vi "Xbox Controller Worker.vi"(8 "Error In":errorcluster, 10 "Events":T2, 11 "Xbox One Controller Ref":T1={"Controller Ref"=refnum, "Event Refnum"=refnum, "Worker Ref"=refnum}) -> (0 "Error Out":errorcluster)   [LabVIEW 2011, in "LVH-Xbox-One-Controller.lvlib"]
uses:
  LVH-Xbox-One-Controller.lvlib
  Type Defs/Events.ctl
  Type Defs/Xbox One Controller Ref.ctl
  Type Defs/Indicators/All Buttons Visual.ctl
  Type Defs/Indicators/A.ctl
  Type Defs/Indicators/B.ctl
  Type Defs/Indicators/X.ctl
  Type Defs/Indicators/Y.ctl
  Type Defs/Indicators/Left Bumper.ctl
  Type Defs/Indicators/Right Bumper.ctl
  Type Defs/Indicators/View.ctl
  Type Defs/Indicators/Menu.ctl
  Type Defs/Indicators/Thumbstick.ctl
  <vilib>/Utility/inputDevices.llb/joystickAcquire.vi
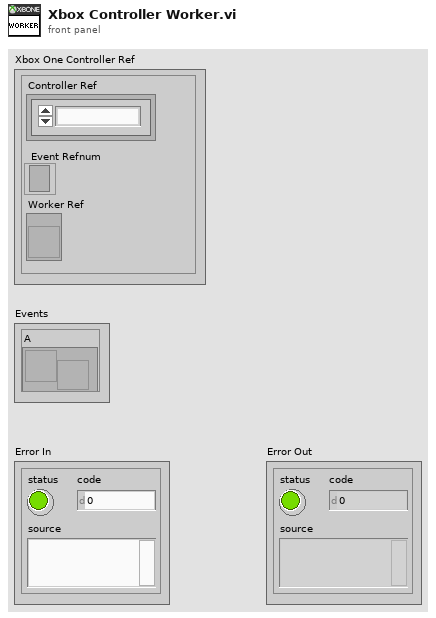
[diagram p1: front panel]
types:
  T1 = typedef "LVH-Xbox-One-Controller.lvlib/Xbox One Controller Ref.ctl" = cluster{"Controller Ref":refnum<k1>, "Event Refnum":refnum<event-registration>, "Worker Ref":refnum<vi>}
  T2 = typedef "LVH-Xbox-One-Controller.lvlib/Events.ctl" = cluster{"A":refnum<user-event>, "B":refnum<user-event>, "X":refnum<user-event>, "Y":refnum<user-event>, "Left Bumper":refnum<user-event>, "Right Bumper":refnum<user-event>, "View":refnum<user-event>, "Menu":refnum<user-event>, "Left Stick":refnum<user-event>, "Right Stick":refnum<user-event>}
  T3 = typedef "LVH-Xbox-One-Controller.lvlib/All Buttons Visual.ctl" = cluster{"A":T4, "B":T5, "X":T6, "Y":T7, "Left Bumper":T8, "Right Bumper":T9, "View Button":T10, "Menu Button":T11, "Left Stick":T12, "Right Stick":T12}
  T4 = typedef "LVH-Xbox-One-Controller.lvlib/A.ctl" = bool
  T5 = typedef "LVH-Xbox-One-Controller.lvlib/B.ctl" = bool
  T6 = typedef "LVH-Xbox-One-Controller.lvlib/X.ctl" = bool
  T7 = typedef "LVH-Xbox-One-Controller.lvlib/Y.ctl" = bool
  T8 = typedef "LVH-Xbox-One-Controller.lvlib/Left Bumper.ctl" = bool
  T9 = typedef "LVH-Xbox-One-Controller.lvlib/Right Bumper.ctl" = bool
  T10 = typedef "LVH-Xbox-One-Controller.lvlib/View.ctl" = bool
  T11 = typedef "LVH-Xbox-One-Controller.lvlib/Menu.ctl" = bool
  T12 = typedef "LVH-Xbox-One-Controller.lvlib/Thumbstick.ctl" = bool
  T13 = cluster{"button 1":bool, "button 2":bool, "button 3":bool, "button 4":bool, "button 5":bool, "button 6":bool, "button 7":bool, "button 8":bool, "button 9":bool, "button 10":bool, "button 11":bool, "button 12":bool, "button 13":bool, "button 14":bool, "button 15":bool, "button 16":bool, "button 17":bool, "button 18":bool, "button 19":bool, "button 20":bool, "button 21":bool, "button 22":bool, "button 23":bool, "button 24":bool, "button 25":bool, "button 26":bool, "button 27":bool, "button 28":bool, "button 29":bool, "button 30":bool, "button 31":bool, "button 32":bool}
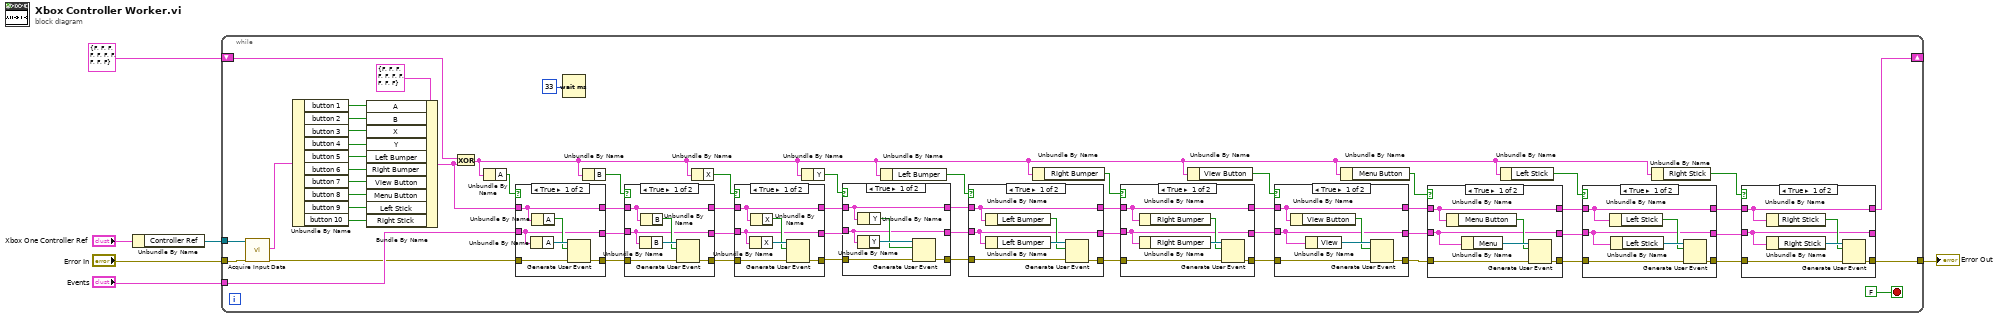
[diagram p0: block diagram]
diagram:
  n1 = Unbundle By Name("Xbox One Controller Ref") -> ("Controller Ref"=w5:refnum<k1>)
  n2 = while {
    tunnel: w5 -> [w66]
    tunnel: "Error In" -> [w65]
    shift-right: [w8] -> _
    shift-left: T3 {"A"=FALSE, "B"=FALSE, "X"=FALSE, "Y"=FALSE, "Left Bumper"=FALSE, "Right Bumper"=FALSE, "View Button"=FALSE, "Menu Button"=FALSE, "Left Stick"=FALSE, "Right Stick"=FALSE} ("Buttons") -> [w52]
    tunnel: "Events" -> [w49]
    tunnel: [w9] -> w1
    stop <- FALSE stop-if-true
    n3 = call-poly <vilib>:"Acquire Input Data.vi"("device ID"=w66, "error in (no error)"=w65) -> ("button info"=w53:T13, "error out"=w48:errorcluster)  [unwired: 13 in, 3 out]
    n4 = Unbundle By Name(w53) -> ("button 1"=w63:bool, "button 2"=w62:bool, "button 3"=w61:bool, "button 4"=w60:bool, "button 5"=w59:bool, "button 6"=w58:bool, "button 7"=w57:bool, "button 8"=w56:bool, "button 9"=w55:bool, "button 10"=w54:bool)
    n5 = Bundle By Name(cluster=T3 {"A"=FALSE, "B"=FALSE, "X"=FALSE, "Y"=FALSE, "Left Bumper"=FALSE, "Right Bumper"=FALSE, "View Button"=FALSE, "Menu Button"=FALSE, "Left Stick"=FALSE, "Right Stick"=FALSE} ("Buttons"), "A"=w63, "B"=w62, "X"=w61, "Y"=w60, "Left Bumper"=w59, "Right Bumper"=w58, "View Button"=w57, "Menu Button"=w56, "Left Stick"=w55, "Right Stick"=w54) -> (w50:T3)
    n6 = Exclusive Or(1:w50, 2:w52) -> (0:w10:T3)
    n7 = Unbundle By Name(w10) -> ("A"=w51:T4)
    n8 = case shown="True" w51 {
      tunnel: [w153 w156] -> w44
      tunnel: w50 -> [w148 w154]
      tunnel: w49 -> [w149 w155]
      tunnel: w48 -> [w150 w156]
      tunnel: [w149 w155] -> w45
      tunnel: [w148 w154] -> w46
      frame True {
        n9 = Unbundle By Name(w149) -> ("A"=w152:refnum<user-event>)
        n10 = Unbundle By Name(w148) -> ("A"=w151:T4)
        n11 = Generate User Event(user event=w152, event data cluster=w151, error in=w150) -> (error out=w153:errorcluster)  [unwired: 1 out]
      }
      frame False {
        # "No Change"
      }
    }
    n12 = Wait (ms)(milliseconds to wait=u32 33) -> ()  [unwired: 1 out]
    n13 = Unbundle By Name(w10) -> ("B"=w47:T5)
    n14 = case shown="True" w47 {
      tunnel: [w144 w147] -> w38
      tunnel: w46 -> [w139 w145]
      tunnel: w45 -> [w140 w146]
      tunnel: w44 -> [w141 w147]
      tunnel: [w140 w146] -> w37
      tunnel: [w139 w145] -> w42
      frame True {
        n15 = Unbundle By Name(w140) -> ("B"=w143:refnum<user-event>)
        n16 = Unbundle By Name(w139) -> ("B"=w142:T5)
        n17 = Generate User Event(user event=w143, event data cluster=w142, error in=w141) -> (error out=w144:errorcluster)  [unwired: 1 out]
      }
      frame False {
        # "No Change"
      }
    }
    n18 = Unbundle By Name(w10) -> ("X"=w34:T6)
    n19 = case shown="True" w34 {
      tunnel: [w135 w138] -> w39
      tunnel: w42 -> [w130 w136]
      tunnel: w37 -> [w131 w137]
      tunnel: w38 -> [w132 w138]
      tunnel: [w131 w137] -> w40
      tunnel: [w130 w136] -> w41
      frame True {
        n20 = Unbundle By Name(w131) -> ("X"=w134:refnum<user-event>)
        n21 = Unbundle By Name(w130) -> ("X"=w133:T6)
        n22 = Generate User Event(user event=w134, event data cluster=w133, error in=w132) -> (error out=w135:errorcluster)  [unwired: 1 out]
      }
      frame False {
        # "No Change"
      }
    }
    n23 = Unbundle By Name(w10) -> ("Y"=w33:T7)
    n24 = case shown="True" w33 {
      tunnel: [w126 w129] -> w29
      tunnel: w41 -> [w121 w127]
      tunnel: w40 -> [w122 w128]
      tunnel: w39 -> [w123 w129]
      tunnel: [w122 w128] -> w36
      tunnel: [w121 w127] -> w35
      frame True {
        n25 = Unbundle By Name(w122) -> ("Y"=w125:refnum<user-event>)
        n26 = Unbundle By Name(w121) -> ("Y"=w124:T7)
        n27 = Generate User Event(user event=w125, event data cluster=w124, error in=w123) -> (error out=w126:errorcluster)  [unwired: 1 out]
      }
      frame False {
        # "No Change"
      }
    }
    n28 = Unbundle By Name(w10) -> ("Left Bumper"=w32:T8)
    n29 = case shown="True" w32 {
      tunnel: [w117 w118] -> w28
      tunnel: w35 -> [w113 w119]
      tunnel: w36 -> [w114 w120]
      tunnel: [w114 w120] -> w26
      tunnel: [w113 w119] -> w31
      tunnel: w29 -> [w112 w118]
      frame True {
        n30 = Unbundle By Name(w113) -> ("Left Bumper"=w115:T8)
        n31 = Unbundle By Name(w114) -> ("Left Bumper"=w116:refnum<user-event>)
        n32 = Generate User Event(user event=w116, event data cluster=w115, error in=w112) -> (error out=w117:errorcluster)  [unwired: 1 out]
      }
      frame False {
        # "No Change"
      }
    }
    n33 = Unbundle By Name(w10) -> ("Right Bumper"=w24:T9)
    n34 = case shown="True" w24 {
      tunnel: [w108 w109] -> w27
      tunnel: w31 -> [w104 w110]
      tunnel: w26 -> [w105 w111]
      tunnel: [w105 w111] -> w25
      tunnel: [w104 w110] -> w30
      tunnel: w28 -> [w103 w109]
      frame True {
        n35 = Unbundle By Name(w104) -> ("Right Bumper"=w106:T9)
        n36 = Unbundle By Name(w105) -> ("Right Bumper"=w107:refnum<user-event>)
        n37 = Generate User Event(user event=w107, event data cluster=w106, error in=w103) -> (error out=w108:errorcluster)  [unwired: 1 out]
      }
      frame False {
        # "No Change"
      }
    }
    n38 = Unbundle By Name(w10) -> ("View Button"=w23:T10)
    n39 = case shown="True" w23 {
      tunnel: [w99 w100] -> w20
      tunnel: w30 -> [w95 w101]
      tunnel: w25 -> [w96 w102]
      tunnel: [w96 w102] -> w21
      tunnel: [w95 w101] -> w22
      tunnel: w27 -> [w94 w100]
      frame True {
        n40 = Unbundle By Name(w95) -> ("View Button"=w97:T10)
        n41 = Unbundle By Name(w96) -> ("View"=w98:refnum<user-event>)
        n42 = Generate User Event(user event=w98, event data cluster=w97, error in=w94) -> (error out=w99:errorcluster)  [unwired: 1 out]
      }
      frame False {
        # "No Change"
      }
    }
    n43 = Unbundle By Name(w10) -> ("Menu Button"=w19:T11)
    n44 = case shown="True" w19 {
      tunnel: [w90 w91] -> w16
      tunnel: w22 -> [w86 w92]
      tunnel: w21 -> [w87 w93]
      tunnel: [w87 w93] -> w17
      tunnel: [w86 w92] -> w18
      tunnel: w20 -> [w85 w91]
      frame True {
        n45 = Unbundle By Name(w86) -> ("Menu Button"=w88:T11)
        n46 = Unbundle By Name(w87) -> ("Menu"=w89:refnum<user-event>)
        n47 = Generate User Event(user event=w89, event data cluster=w88, error in=w85) -> (error out=w90:errorcluster)  [unwired: 1 out]
      }
      frame False {
        # "No Change"
      }
    }
    n48 = Unbundle By Name(w10) -> ("Left Stick"=w12:T12)
    n49 = case shown="True" w12 {
      tunnel: [w81 w82] -> w13
      tunnel: w18 -> [w77 w83]
      tunnel: w17 -> [w78 w84]
      tunnel: [w78 w84] -> w14
      tunnel: [w77 w83] -> w15
      tunnel: w16 -> [w76 w82]
      frame True {
        n50 = Unbundle By Name(w77) -> ("Left Stick"=w79:T12)
        n51 = Unbundle By Name(w78) -> ("Left Stick"=w80:refnum<user-event>)
        n52 = Generate User Event(user event=w80, event data cluster=w79, error in=w76) -> (error out=w81:errorcluster)  [unwired: 1 out]
      }
      frame False {
        # "No Change"
      }
    }
    n53 = Unbundle By Name(w10) -> ("Right Stick"=w11:T12)
    n54 = case shown="True" w11 {
      tunnel: [w72 w73] -> w9
      tunnel: w15 -> [w68 w74]
      tunnel: w14 -> [w69 w75]
      tunnel: [w69 w75] -> _
      tunnel: [w68 w74] -> w8
      tunnel: w13 -> [w67 w73]
      frame True {
        n55 = Unbundle By Name(w68) -> ("Right Stick"=w70:T12)
        n56 = Unbundle By Name(w69) -> ("Right Stick"=w71:refnum<user-event>)
        n57 = Generate User Event(user event=w71, event data cluster=w70, error in=w67) -> (error out=w72:errorcluster)  [unwired: 1 out]
      }
      frame False {
        # "No Change"
      }
    }
  }
  "Error Out" <- w1
